vi "PCU_DisConnect.vi"(3 "error in (no error)":errorcluster, 5 ".NET Reference in":refnum<k24>) -> (0 "error out":errorcluster, 2 "Reference out":refnum<k24>)   [LabVIEW 2017]
uses:
  LV_IL_Sample/DLL/InstrumentDLL.dll
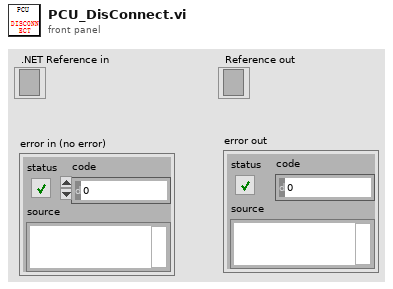
[diagram p1: front panel]
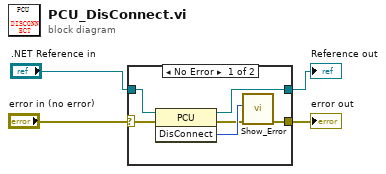
[diagram p0: block diagram]
diagram:
  n1 = case shown="No Error" "error in (no error)" {
    selector: "error in (no error)" -> [w8 w12]
    tunnel: [w5 w12] -> w4
    tunnel: ".NET Reference in" -> [w10 w11]
    tunnel: [w9 w11] -> w2
    frame No Error {
      n2 = invoke on="调用节点" class="PCU" method="DisConnect"(reference=w10, error in=w8) -> (reference out=w9:refnum<k24>, error out=w6:errorcluster, "DisConnect"=w7:i32)  [unwired: 1 in]
      n3 = call "Show_Error.vi"("error in (no error)"=w6, "Error"=w7) -> ("error out"=w5:errorcluster)  [unwired: 9 in]
    }
    frame Error {
    }
  }
  "error out" <- w4
  "Reference out" <- w2
